vi "UDT_ErrorMonitorModule_ErrorPostRun.vi"() -> (3 "Unit Test Framework Results":T1)   [LabVIEW 2017]
doc: "Use this template to create a user-defined test VI. Define your test requirements and wire the results to the <b>Result (Test)</b> control. Do not modify the <b>Unit Test Framework Results</b> indicator."
uses:
  <vilib>/utf/common/utf_test_result_troll.ctl
  <vilib>/utf/common/utf_test_result.ctl
  <vilib>/utf/common/utf_test_result_failure.ctl
  <vilib>/utf/common/utf_test_comparison_operators.ctl
  <vilib>/utf/common/utf_vi_tag.ctl
  RT/ErrorMonitor/Queue/TypeDefs/queueFGVState.ctl
  RT/ErrorMonitor/Queue/TypeDefs/message.ctl
  <vilib>/Control Software Solutions Ltd/UTF Helper/SubVIs/UTF Variant Equals.vi
  <vilib>/Control Software Solutions Ltd/UTF Helper/Unit Test Helper.lvlib
  RT/ErrorMonitor/ErrorMonitor.lvlib
  <vilib>/utf/NI_UnitTestFramework.lvlib
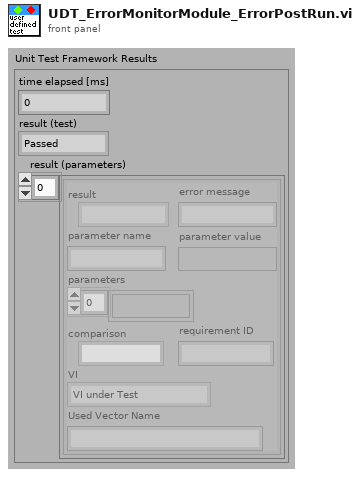
[diagram p1: front panel]
types:
  T1 = typedef "NI_UnitTestFramework.lvlib/utf_test_result_troll.ctl" = cluster{"time elapsed [ms]":u32, "result (test)":T2, "result (parameters)":T3[]}
  T2 = typedef "NI_UnitTestFramework.lvlib/utf_test_result.ctl" = enum16{"Passed", "Failed", "Error", "Skipped", "Not Processed"}
  T3 = typedef "NI_UnitTestFramework.lvlib/utf_test_result_failure.ctl" = cluster{"result":T2, "error message":string, "parameter name":string, "parameter value":variant, "parameters":variant[], "comparison":T4, "requirement ID":string, "VI":T5, "Used Vector Name":string}
  T4 = typedef "NI_UnitTestFramework.lvlib/utf_test_comparison_operators.ctl" = enum16{"=", "!=", ">", ">=", "<", "<=", "range", "symmetric tolerance", "asymmetric tolerance", "string contains", "string not contain", "array size", "string length", "array range", "by element", "array range (limit array)", "user-defined", "array contains", "array not contain", "vector length", "= (elm)", "!= (elm)", "= (case insensitive)", "!= (case insensitive)"}
  T5 = typedef "NI_UnitTestFramework.lvlib/utf_vi_tag.ctl" = enum16{"Setup VI", "VI under Test", "Teardown VI"}
  T6 = typedef "ErrorMonitor.lvlib/message.ctl" = cluster{"calling module":string, "message":string, "Data":variant}
  T7 = typedef "ErrorMonitor.lvlib/queueFGVState.ctl" = enum16{"obtain", "enqueue low priority", "enqueue high priority", "dequeue", "release"}
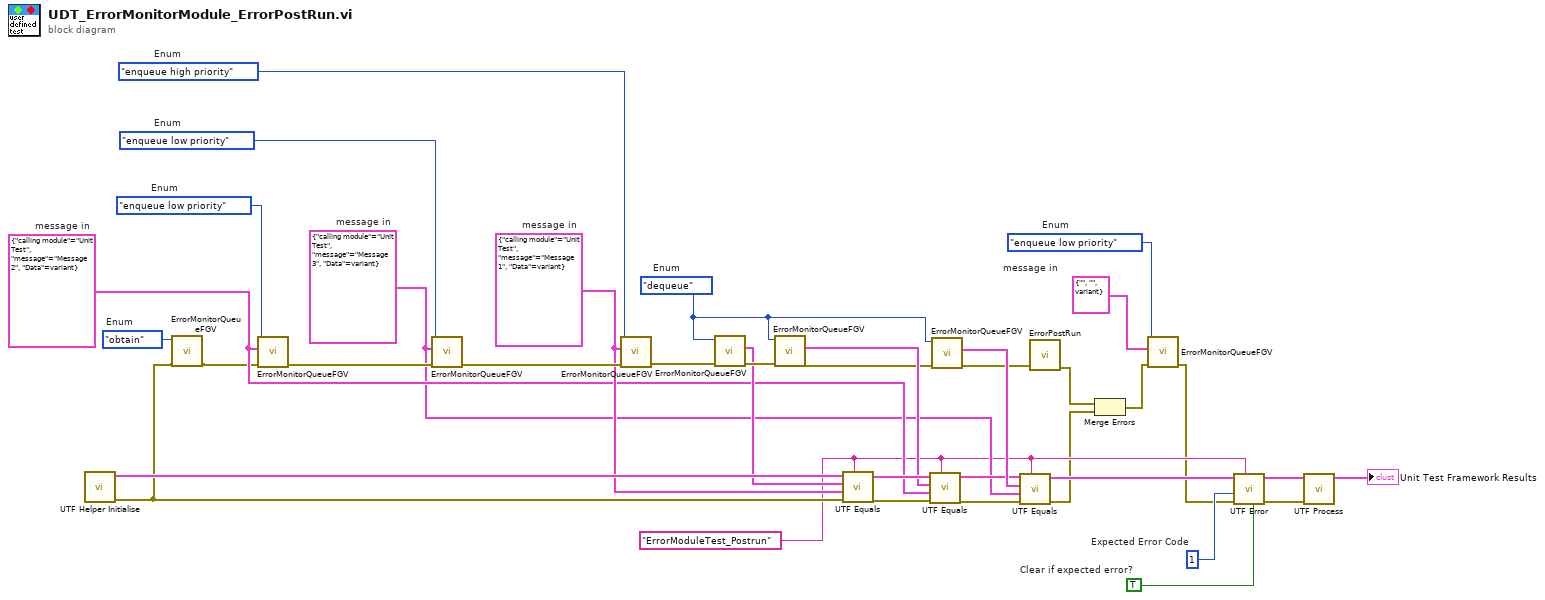
[diagram p0: block diagram]
diagram:
  w6 = TRUE  # Clear if expected error?
  w7 = 1  # Expected Error Code
  w12 = T6 {"calling module"="", "message"="", "Data"=variant}  # message in
  w13 = queueFGVState."enqueue low priority"  # Enum
  w15 = queueFGVState."obtain"  # Enum
  w8 = "ErrorModuleTest_Postrun"
  w22 = queueFGVState."dequeue"  # Enum
  w31 = T6 {"calling module"="Unit Test", "message"="Message 1", "Data"=variant}  # message in
  w18 = T6 {"calling module"="Unit Test", "message"="Message 3", "Data"=variant}  # message in
  w24 = T6 {"calling module"="Unit Test", "message"="Message 2", "Data"=variant}  # message in
  w34 = queueFGVState."enqueue high priority"  # Enum
  w36 = queueFGVState."enqueue low priority"  # Enum
  w37 = queueFGVState."enqueue low priority"  # Enum
  n1 = call <vilib>:"UTF Helper Initialise.vi"() -> ("error out"=w17:errorcluster, "results array"=w32:T3[])  [unwired: 10 in]
  n2 = call "ErrorMonitorQueueFGV.vi"("error in (no error)"=w17, "Enum"=w15) -> ("error out"=w16:errorcluster)  [unwired: 8 in, 1 out]
  n3 = call "ErrorMonitorQueueFGV.vi"("error in (no error)"=w16, "message in"=w24, "Enum"=w37) -> ("error out"=w35:errorcluster)  [unwired: 7 in, 1 out]
  n4 = call "ErrorMonitorQueueFGV.vi"("error in (no error)"=w35, "message in"=w18, "Enum"=w36) -> ("error out"=w33:errorcluster)  [unwired: 7 in, 1 out]
  n5 = call "ErrorMonitorQueueFGV.vi"("error in (no error)"=w33, "message in"=w31, "Enum"=w34) -> ("error out"=w30:errorcluster)  [unwired: 7 in, 1 out]
  n6 = call "ErrorMonitorQueueFGV.vi"("error in (no error)"=w30, "Enum"=w22) -> ("error out"=w27:errorcluster, "message out"=w26:T6)  [unwired: 8 in]
  n7 = call "ErrorMonitorQueueFGV.vi"("error in (no error)"=w27, "Enum"=w22) -> ("error out"=w23:errorcluster, "message out"=w25:T6)  [unwired: 8 in]
  n8 = call-poly <vilib>:"UTF Equals.vi"("Parameter Name"=w8, "error in (no error)"=w17, "Test Value"=w31, "Input"=w26, "Input Results"=w32) -> ("error out"=w29:errorcluster, "Output Results"=w28:T3[])  [unwired: 5 in]
  n9 = call-poly <vilib>:"UTF Equals.vi"("Parameter Name"=w8, "error in (no error)"=w29, "Test Value"=w24, "Input"=w25, "Input Results"=w28) -> ("error out"=w19:errorcluster, "Output Results"=w20:T3[])  [unwired: 5 in]
  n10 = call "ErrorMonitorQueueFGV.vi"("error in (no error)"=w23, "Enum"=w22) -> ("error out"=w14:errorcluster, "message out"=w21:T6)  [unwired: 8 in]
  n11 = call-poly <vilib>:"UTF Equals.vi"("Parameter Name"=w8, "error in (no error)"=w19, "Test Value"=w18, "Input"=w21, "Input Results"=w20) -> ("error out"=w4:errorcluster, "Output Results"=w10:T3[])  [unwired: 5 in]
  n12 = call "ErrorPostRun.vi"("error in (no error)"=w14) -> ("error out"=w5:errorcluster)  [unwired: 10 in]
  n13 = Merge Errors(w5, w4) -> (w3:errorcluster)
  n14 = call "ErrorMonitorQueueFGV.vi"("error in (no error)"=w3, "message in"=w12, "Enum"=w13) -> ("error out"=w2:errorcluster)  [unwired: 7 in, 1 out]
  n15 = call <vilib>:"UTF Error.vi"("Clear if expected error?"=w6, "Parameter Name"=w8, "error in (no error)"=w2, "Expected Error Code"=w7, "Input Results"=w10) -> ("error out"=w11:errorcluster, "Output Results"=w9:T3[])  [unwired: 5 in]
  n16 = call <vilib>:"UTF Process.vi"("error in (no error)"=w11, "results array"=w9) -> ("Unit Test Framework Results"=→"Unit Test Framework Results":T1)  [unwired: 9 in]
